vi "Volume ROI entry user dialogue handler.vi"(7 "Center around clicked pixel (F)":bool, 8 "error in (no error)":errorcluster, 11 "New coordinates":i32[](array[numeric])) -> (0 "error IO":errorcluster, 1 "Cancelled":bool, 3 "ROIs Info []":T1[](array[typedef]) {"Zoom" min=1.0 max=10.0 step=0.10000000149011612})   [LabVIEW 2013]
uses:
  Typedefs/ROI spec.ctl
  Typedefs/ROI ID Enum.ctl
  ROI Entry screen/Globals/gl_ROI Entry UI globals.vi
panel:
  out "Modified coordinates":i32[](array[numeric])
  # "Tick the box below if you want to specify a volume from the rectangular shaped you have drawn and enter select the two z--planes between which the volume should be created."
  # "X1\nY1\nX2\nY2"
  # "X1\nY1\nX2\nY2"
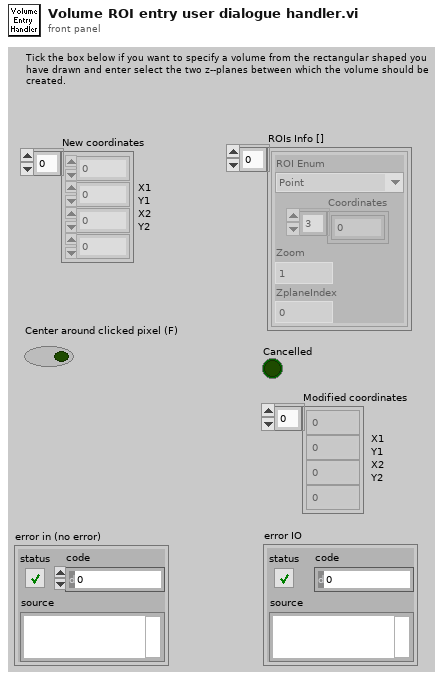
[diagram p1: front panel]
types:
  T1 = typedef "ROI spec.ctl" = cluster{"Coordinates":i32[], "Zoom":dbl, "ROI Enum":T2, "ZplaneIndex":i32}
  T2 = typedef "ROI ID Enum.ctl" = enum16{"Point", "MiniScan", "Comp. MiniScan", "Rectangle", "Comp. volume", "Arb. plane point"}
  T3 = typedef "ROI entry screen ctrl refs cluster.ctl" = cluster{"Done button":refnum<vi>, "Imaging button":refnum<vi>, "Acquisition button":refnum<vi>, "POI dwell time (us)":refnum<vi>, "Scan dwell time per pixel (us)":refnum<vi>, "# of planes":refnum<vi>, "Zoom":refnum<vi>, "Equal size":refnum<vi>, "Channel":refnum<vi>, "Image Display":refnum<vi>, "Z-Plane Selector":refnum<vi>, "Number of lines left":refnum<vi>, "Z-stack folder path":refnum<vi>, "POI Density":refnum<vi>, "Arb Plane Entry":refnum<vi>, "Whole plane":refnum<vi>, "Clear Last":refnum<vi>, "Clear All":refnum<vi>, "Trial Length (sec)":refnum<vi>, "Palette Type":refnum<vi>, "Intensity slider":refnum<vi>, "# POI":refnum<vi>, "Max Z Proj":refnum<vi>, "Zplane ind":refnum<vi>, "Wavelength (nm)":refnum<vi>, "Number of Trials":refnum<vi>, "Funct stim.trig.enable":refnum<vi>, "Funct stim.trig.delay (s)":refnum<vi>, "Line Mode":refnum<vi>, "Step size (µm)":refnum<vi>, "ROI move mode":refnum<vi>, "Cool-down time (s)":refnum<vi>, "Enable cool-down time":refnum<vi>, "Motor Z ind. (um)":refnum<vi>, "AOL Z ind. (um)":refnum<vi>}
  T4 = typedef "ROI input mode.ctl" = enum16{"Unspecified", "Point-Line-Plane", "Volume"}
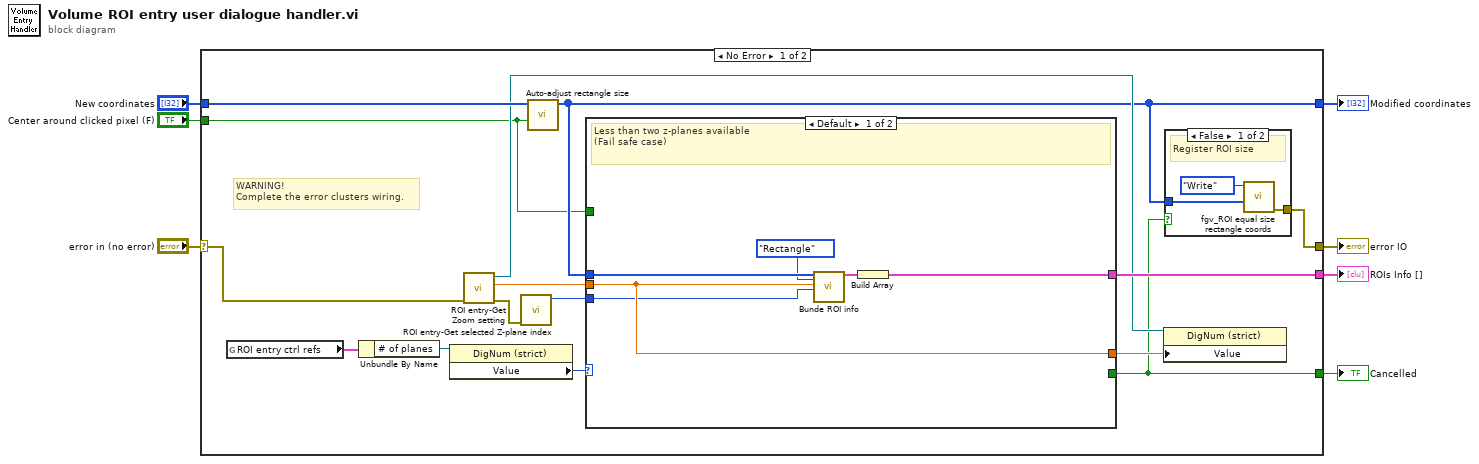
[diagram p0: block diagram]
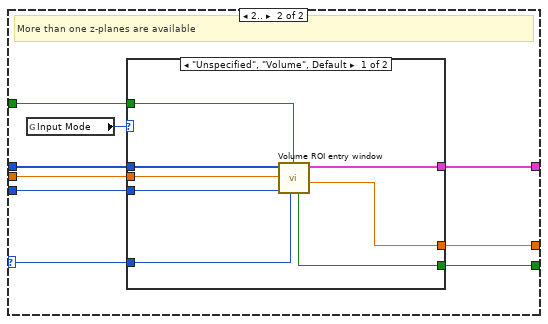
[diagram p3: hidden frame]
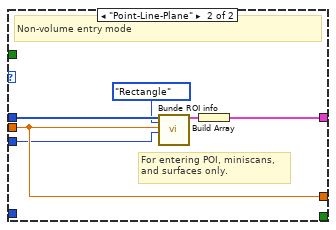
[diagram p4: hidden frame]
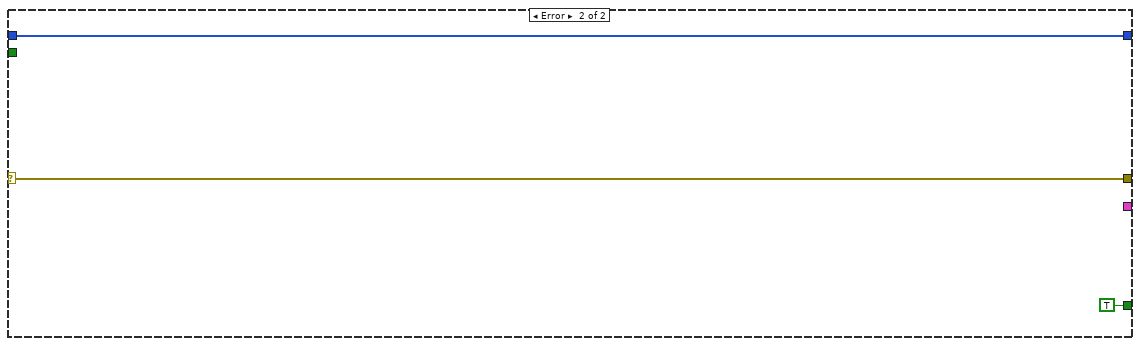
[diagram p5: hidden frame]
diagram:
  n1 = case shown="No Error" "error in (no error)" {
    selector: "error in (no error)" -> [w9 w57]
    tunnel: [w22 _] -> w7
    tunnel: "New coordinates" -> [w21 w55]
    tunnel: [w13 w55] -> w5
    tunnel: [w12 TRUE ("Cancelled")] -> w4
    tunnel: [w10 w57] -> w2
    tunnel: "Center around clicked pixel (F)" -> [w8 _]
    frame No Error {
      # "WARNING!\nComplete the error clusters wiring."
      n2 = global read "gl_ROI Entry UI globals.vi" "ROI entry ctrl refs"() -> (w19:T3)
      n3 = Unbundle By Name(w19) -> ("# of planes"=w20:refnum<vi>)
      n4 = property class="DigNum (strict)"(reference=w20) -> ("Value"=w18:i32)  [unwired: 1 in, 2 out]
      n5 = call "ROI entry-Get Zoom setting.vi"("error in (no error)"=w9) -> ("error out"=w11:errorcluster, "Zoom Value"=w16:dbl, "Zoom control ref"=w15:refnum<vi>)  [unwired: 8 in]
      n6 = call "ROI entry-Get selected Z-plane index.vi"("error in (no error)"=w11) -> ("Z-plane selector (index)"=w14:i32)  [unwired: 9 in, 1 out]
      n7 = call "Auto-adjust rectangle size.vi"("Center around clicked pixel (F)"=w8, "New Coordinates"=w21) -> ("Modified coordinates"=w13:i32[])  [unwired: 9 in]
      n8 = case shown="Default" w18 {
        selector: w18 -> [_ w37]
        tunnel: [w31 w38] -> w22
        tunnel: w13 -> [w30 w40]
        tunnel: w14 -> [w26 w39]
        tunnel: [_ w36] -> w12
        tunnel: w16 -> [w28 w34]
        tunnel: [w28 w33] -> w17
        tunnel: w8 -> [_ w32]
        frame Default {
          # "Less than two z-planes available\n(Fail safe case)"
          n9 = call "Bunde ROI info.vi"("ROI Coordinates"=w30, "ROI Enum"=ROI_ID_Enum."Rectangle", "Zoom"=w28, "ZplaneIndex"=w26) -> ("ROI Info"=w29:T1)  [unwired: 15 in]
          n10 = Build Array(w29) -> (w31:T1[])
        }
        frame 2.. {
          # "More than one z-planes are available"
          n11 = global read "gl_ROI Entry UI globals.vi" "Input Mode"() -> (w35:T4)
          n12 = case shown="\"Unspecified\", \"Volume\", Default" w35 {
            tunnel: w40 -> [w48 w53]
            tunnel: w39 -> [w47 w49]
            tunnel: [w46 w54] -> w38
            tunnel: w37 -> [w45 _]
            tunnel: [w44 _] -> w36
            tunnel: w34 -> [w43 w51]
            tunnel: [w42 w51] -> w33
            tunnel: w32 -> [w41 _]
            frame "Unspecified", "Volume", Default {
              n13 = call "Volume ROI entry window.vi"("# of planes"=w45, "Do not initialise selector values"=w41, "ZplaneIndex (zero based)"=w47, "Zoom (in)"=w43, "Coordinates"=w48) -> ("Zoom (out)"=w42:dbl, "ROIs Info []"=w46:T1[], "Cancelled"=w44:bool)  [unwired: 4 in]
            }
            frame "Point-Line-Plane" {
              # "For entering POI, miniscans,\nand surfaces only."
              # "Non-volume entry mode"
              n14 = call "Bunde ROI info.vi"("ROI Coordinates"=w53, "ROI Enum"=ROI_ID_Enum."Rectangle", "Zoom"=w51, "ZplaneIndex"=w49) -> ("ROI Info"=w52:T1)  [unwired: 15 in]
              n15 = Build Array(w52) -> (w54:T1[])
            }
          }
        }
      }
      n16 = property class="DigNum (strict)"(reference=w15, "Value"=w17) -> ()  [unwired: 1 in, 2 out]
      n17 = case shown="False" w12 {
        tunnel: w13 -> [w25 _]
        tunnel: [w23 _] -> w10
        frame False {
          # "Register ROI size"
          n18 = call "fgv_ROI equal size rectangle coords.vi"("New Rectangle Coordinates"=w25, "Function"=enum16{"Intialize", "Write", "Read", "Clear"}."Write") -> ("error out"=w23:errorcluster)  [unwired: 8 in, 1 out]
        }
        frame True {
        }
      }
    }
    frame Error {
    }
  }
  "ROIs Info []" <- w7
  "Cancelled" <- w4
  "Modified coordinates" <- w5
  "error IO" <- w2
